vi "getLocation.vi"(8 "error in (no error)":errorcluster, 11 "Cell in":refnum<class "Cell.lvclass">) -> (0 "error out":errorcluster, 2 "Location":cluster{"X":dbl, "Y":dbl}, 3 "Cell out":refnum<class "Cell.lvclass">)   [LabVIEW 2009, in "Cell.lvclass"]
uses:
  Cell.lvclass
  Cell.lvclass/Cell.ctl
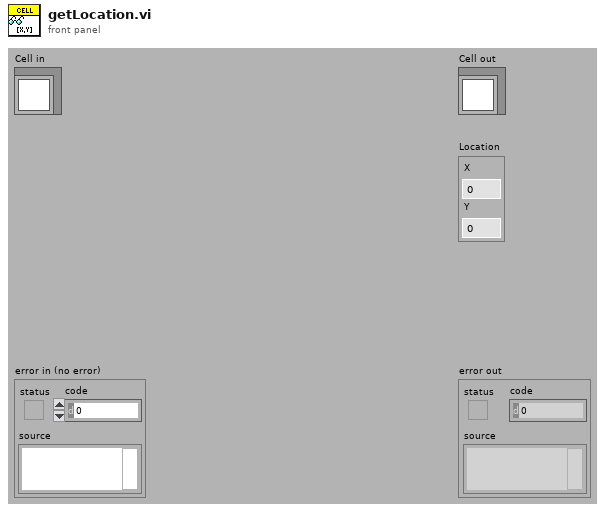
[diagram p1: front panel]
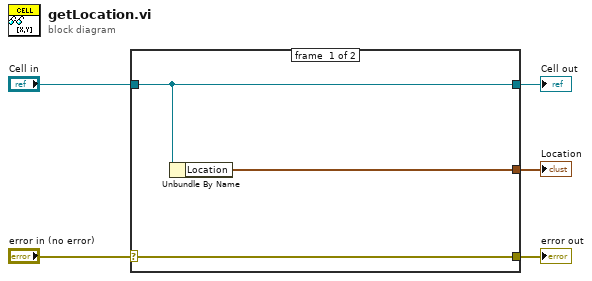
[diagram p0: block diagram]
diagram:
  n1 = case shown="No Error" "error in (no error)" {
    selector: "error in (no error)" -> [w8 w9]
    tunnel: [w8 w9] -> w4
    tunnel: [w7 w10] -> w2
    tunnel: "Cell in" -> [w7 w10]
    tunnel: [w6 _] -> w1
    frame #0 {
      n2 = Unbundle By Name(w7) -> ("Location"=w6:cluster{"X":dbl, "Y":dbl})
    }
    frame #1 {
    }
  }
  "error out" <- w4
  "Cell out" <- w2
  "Location" <- w1
